vi "ExDriver.vi"(4 "Error In":errorcluster, 7 "Command":string) -> (0 "Error Out":errorcluster, 3 "Response":string)   [LabVIEW 2018]
uses:
  MOKO_LabViewLibrary/MokoLowLevel/MokoLowLovelControl/MLLC_DriverName.ctl
  MOKO_LabViewLibrary/MokoLowLevel/MokoLowLovelControl/MLLC_ConnectCluster.ctl
  MOKO_LabViewLibrary/MokoLowLevel/MokoLowLovelControl/MLLC_InterfaceType.ctl
  MOKO_LabViewLibrary/MokoLowLevel/MokoLowLovelControl/MLLC_OpenedSession.ctl
  MOKO_LabViewLibrary/MokoLowLevel/MokoLowLovelControl/MLLC_InterfaceSettings.ctl
  MOKO_LabViewLibrary/MokoLowLevel/MokoLowLovelControl/MLLC_InterfaceKind.ctl
  MOKO_LabViewLibrary/MokoLowLevel/MokoLowLovelControl/MLLC_Request.ctl
  MOKO_LabViewLibrary/MokoLowLevel/MokoLowLovelControl/MLLC_ResponseInit.ctl
panel:
  in  "Response Init":T1="43B"
  in  "Request":T2="ID"
  in  "Settings":T8={"Saved Data"=variant, "Data"={"Connect"={"InterfaceType"=enum."VISA", "OpenedSession"="", "InterfaceSettings"={"Interface"=enum."RS232", "EOS 4 read"=enum."LF (\\n)", "EOS 4 write"=enum."LF (\\n)", "TMO, ms"=10000, "Sett"=variant(cluster{"Baud Rate":u32, "Data Bits":u16, "Parity":u16, "Stop Bits":u16, "Flow Control":u16, "Eho":bool} {"Baud Rate"=75, "Data Bits"=0, "Parity"=0, "Stop Bits"=0, "Flow Control"=0, "Eho"=FALSE})}}, "Values"={"Value"=0.0}}}
  in  "Error Code":u32
  in  "Driver Name":T9="ExDriver"
  in  "Mode":T10(ring)
  # "ExDriver"
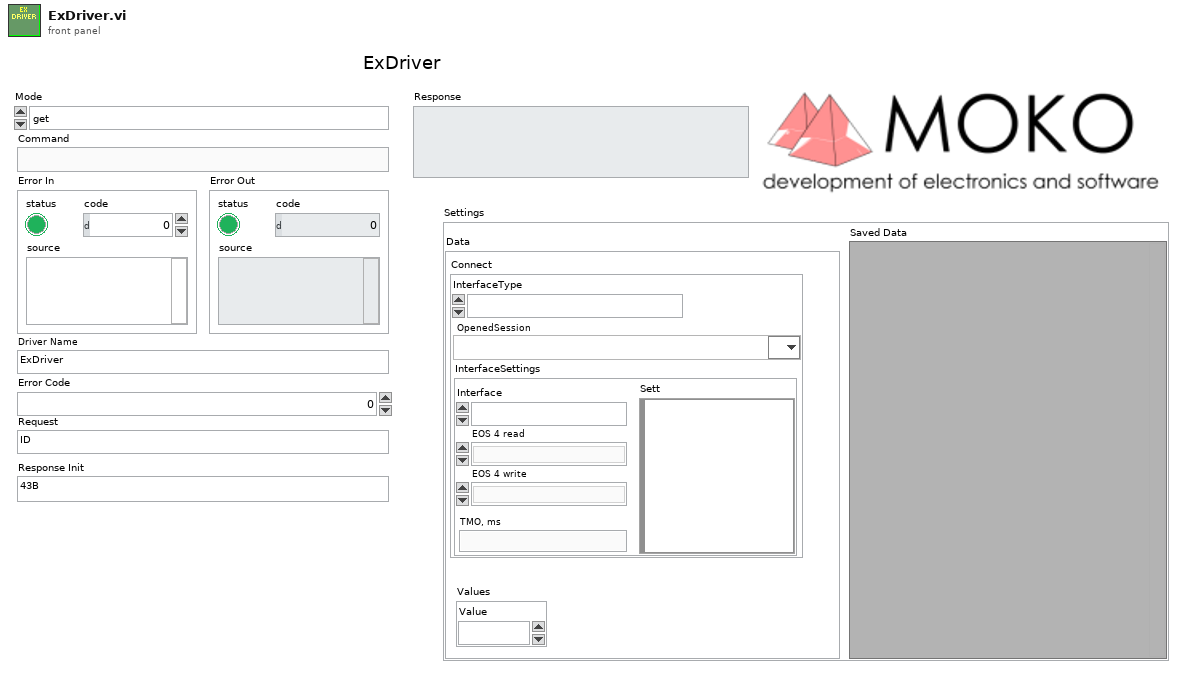
[diagram p1: front panel]
types:
  T1 = typedef "MLLC_ResponseInit.ctl" = string
  T2 = typedef "MLLC_Request.ctl" = string
  T3 = typedef "MLLC_ConnectCluster.ctl" = cluster{"InterfaceType":T4, "OpenedSession":T5, "InterfaceSettings":T6}
  T4 = typedef "MLLC_InterfaceType.ctl" = enum16{"VISA", "Prologix USB-GPIB"}
  T5 = typedef "MLLC_OpenedSession.ctl" = refnum<visa-resource-name>
  T6 = typedef "MLLC_InterfaceSettings.ctl" = cluster{"Interface":T7, "EOS 4 read":enum16{"Default (=EOS 4 write)", "CR (\\r)", "LF (\\n)", "None"}, "EOS 4 write":enum16{"CR+LF (\\r\\n)", "CR (\\r)", "LF (\\n)", "None"}, "TMO, ms":i32, "Sett":variant}
  T7 = typedef "MLLC_InterfaceKind.ctl" = enum16{"RS232", "GPIB", "USB", "Ethernet", "another"}
  T8 = cluster{"Saved Data":variant, "Data":cluster{"Connect":T3, "Values":cluster{"Value":dbl}}}
  T9 = typedef "MLLC_DriverName.ctl" = string
  T10 = enum16{"get", "set", "close", "Init", "Check", "ID"}
  T11 = cluster{"Connect":T3, "Values":cluster{"Value":dbl}}
  T12 = typedef "MLLC_Mode.ctl" = enum16{"get", "set", "close", "Init", "Check"}
  T13 = typedef "MLLC_Error.ctl" = errorcluster
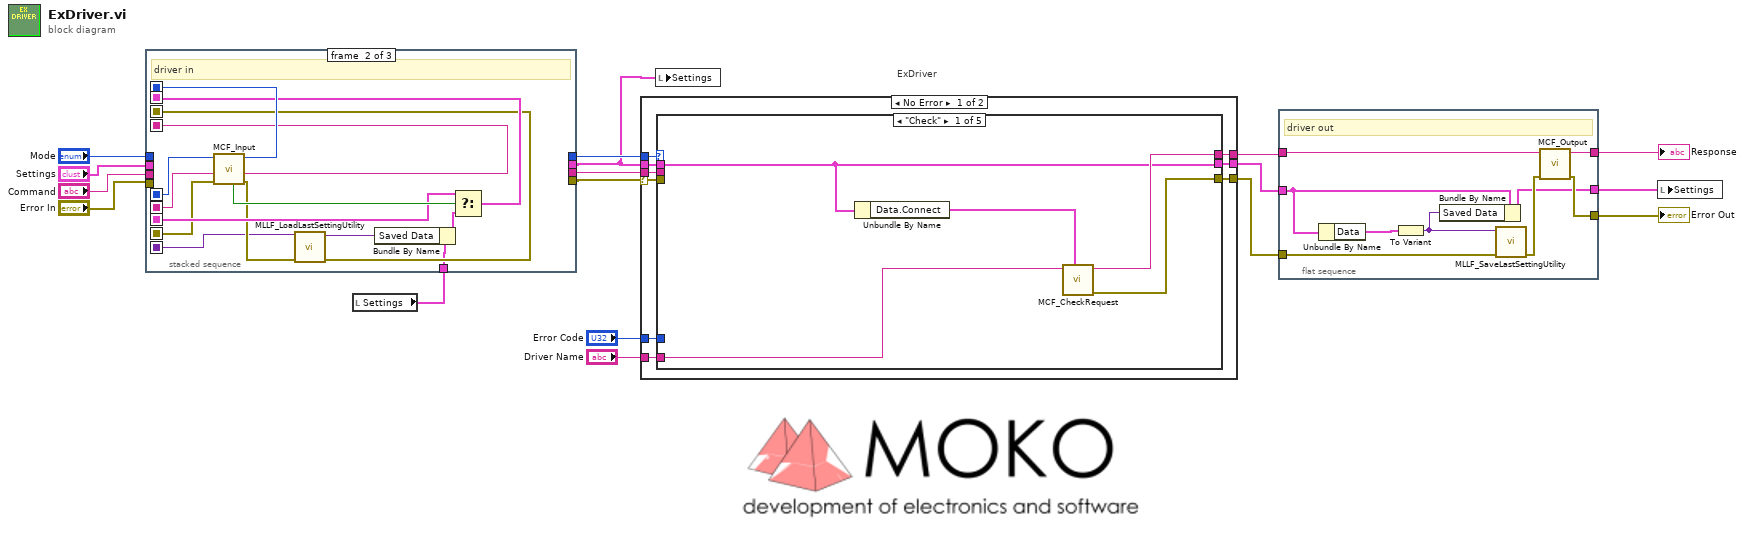
[diagram p0: block diagram]
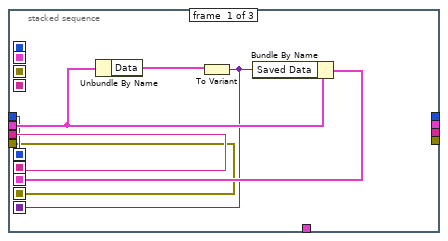
[diagram p2: hidden frame]
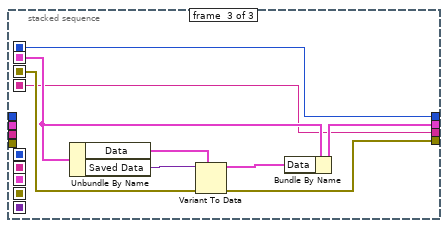
[diagram p3: hidden frame]
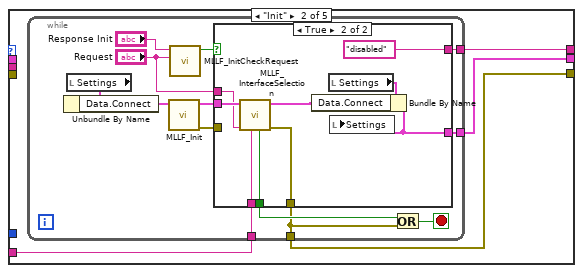
[diagram p4: hidden frame]
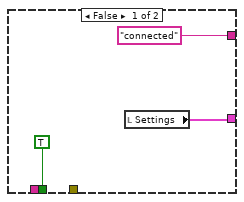
[diagram p5: hidden frame]
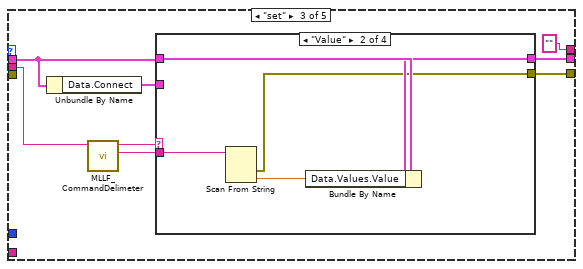
[diagram p6: hidden frame]
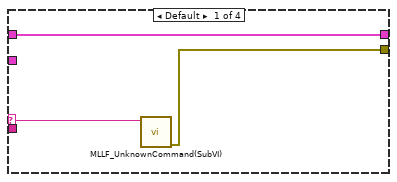
[diagram p7: hidden frame]
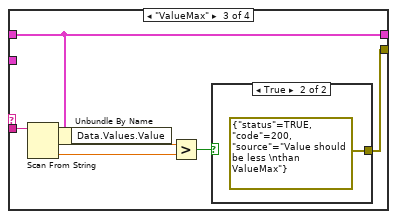
[diagram p8: hidden frame]
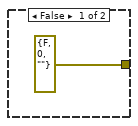
[diagram p9: hidden frame]
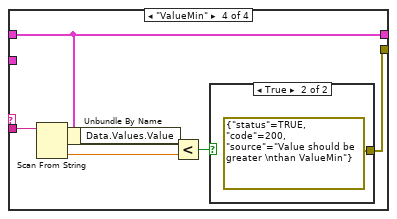
[diagram p10: hidden frame]
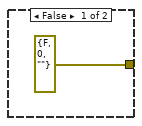
[diagram p11: hidden frame]
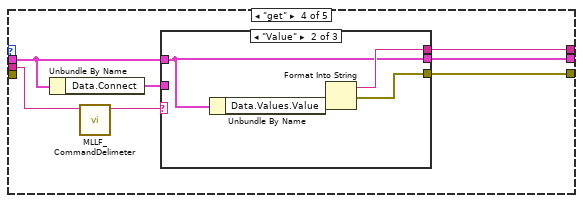
[diagram p12: hidden frame]
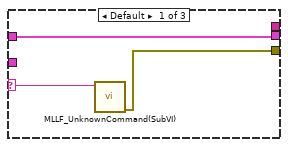
[diagram p13: hidden frame]
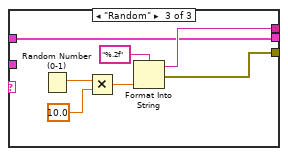
[diagram p14: hidden frame]
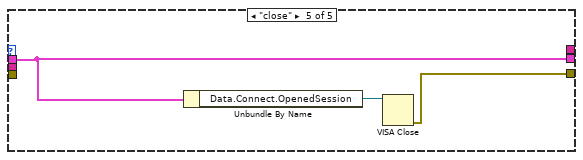
[diagram p15: hidden frame]
diagram:
  # "ExDriver"
  n1 = local read "Settings"() -> (w9:T8)
  n2 = stacked-sequence {
    seq-local: [w20 _ _] -> [_ w36 _]
    seq-local: [w19 _ _] -> [_ w37 _]
    seq-local: [w22 _ _] -> [_ w32 _]
    seq-local: [w18 _ _] -> [_ w31 _]
    seq-local: [w21 _ _] -> [_ w27 _]
    seq-local: [_ w28 _] -> [_ _ w44]
    seq-local: [_ w38 _] -> [_ _ w41]
    seq-local: [_ w35 _] -> [_ _ w40]
    seq-local: [_ w34 _] -> [_ _ w45]
    tunnel: "Command" -> [w20 _ _]
    tunnel: "Mode" -> [w19 _ _]
    tunnel: "Error In" -> [w18 _ _]
    tunnel: "Settings" -> [w23 _ _]
    tunnel: w9 -> [_ w26 _]
    tunnel: [_ _ w40] -> w5
    tunnel: [_ _ w43] -> w6
    tunnel: [_ _ w42] -> w4
    tunnel: [_ _ w41] -> w7
    frame #0 {
      n3 = Unbundle By Name(w23) -> ("Data"=w24:T11)
      n4 = To Variant(anything=w24) -> (Variant=w21:variant)
      n5 = Bundle By Name(cluster=w23, "Saved Data"=w21) -> (w22:T8)
    }
    frame #1 {
      # "driver in"
      n6 = call "MCF_Input.vi"("Error In"=w31, "Command in"=w36, "Mode in"=w37) -> ("Error Out"=w30:errorcluster, "Command out"=w35:string, "Mode out"=w38:T12, "Boolean"=w33:bool)  [unwired: 5 in]
      n7 = call "MLLF_LoadLastSettingUtility.vi"("Error In"=w30, "Save data in"=w27) -> ("Error Out"=w28:errorcluster, "Save data out"=w25:variant)  [unwired: 8 in]
      n8 = Bundle By Name(cluster=w26, "Saved Data"=w25) -> (w29:T8)
      n9 = Select(t=w32, s=w33, f=w29) -> (s? t:f=w34:T8)
    }
    frame #2 {
      n10 = Unbundle By Name(w45) -> ("Data"=w46:T11, "Saved Data"=w39:variant)
      n11 = Variant To Data(error in=w44, type=w46, Variant=w39) -> (data=w47:T11, error out=w42:errorcluster)
      n12 = Bundle By Name(cluster=w45, "Data"=w47) -> (w43:T8)
    }
  }
  n13 = case shown="No Error" w4 {
    selector: w4 -> [w52 w148]
    tunnel: [w54 w148] -> w13
    tunnel: w7 -> [w56 _]
    tunnel: [w55 _] -> w15
    tunnel: w5 -> [w53 _]
    tunnel: w6 -> [w49 w147]
    tunnel: "Error Code" -> [w51 _]
    tunnel: "Driver Name" -> [w50 _]
    tunnel: [w48 w147] -> w14
    frame No Error {
      n14 = case shown="\"Check\"" w56 {
        tunnel: [w60 w63 "" ("Output String") w123 _] -> w55
        tunnel: [w59 w65 w91 w124 w145] -> w54
        tunnel: w53 -> [_ _ w94 w126 _]
        tunnel: w52 -> [_ _ _ _ _]
        tunnel: w51 -> [_ _ _ _ _]
        tunnel: w50 -> [w61 w62 _ _ _]
        tunnel: w49 -> [w58 _ w98 w129 w144]
        tunnel: [w58 w64 w97 w128 w144] -> w48
        frame "Check" {
          # "Проверка подленности пользователя в соответствии с протоколом MD5."
          n15 = Unbundle By Name(w58) -> ("Data.Connect"=w57:T3)
          n16 = call "MCF_CheckRequest.vi"("Permanent data.Connect"=w57, "Driver Name"=w61) -> ("Error Out"=w59:errorcluster, "Output String"=w60:string)  [unwired: 8 in]
        }
        frame "Init" {
          # "Тут проходит инициализация оборудования"
          n17 = while {
            tunnel: [w77] -> w65
            tunnel: w62 -> [w70]
            tunnel: [w74] -> w64
            tunnel: [w71] -> w63
            stop <- w76 stop-if-true
            n18 = local read "Settings"() -> (w75:T8)
            n19 = Unbundle By Name(w75) -> ("Data.Connect"=w73:T3)
            n20 = call "MLLF_Init.vi"("DriverConnect in"=w73) -> ("Error Out"=w67:errorcluster, "DriverConnect out"=w72:T3)  [unwired: 7 in]
            n21 = call "MLLF_InitCheckRequest.vi"("Answer"="Request", "Response Init"="Response Init") -> ("Design"=w68:bool)  [unwired: 6 in, 3 out]
            n22 = case shown="True" w68 {
              tunnel: w72 -> [_ w89]
              tunnel: [TRUE w85] -> w78
              tunnel: [_ w90] -> w77
              tunnel: [w80 w86] -> w74
              tunnel: ["connected" "disabled"] -> w71
              tunnel: w70 -> [_ w83]
              tunnel: w67 -> [_ _]
              tunnel: "Request" -> [_ w82]
              frame False {
                n23 = local read "Settings"() -> (w80:T8)
              }
              frame True {
                n24 = call "MLLF_InterfaceSelection.vi"("Driver Name"=w83, "Answer:"=w82, "DriverConnect in"=w89) -> ("error out"=w90:T13, "DriverConnect out"=w88:T3, "stop init?"=w85:bool)  [unwired: 4 in, 2 out]
                n25 = local read "Settings"() -> (w87:T8)
                n26 = Bundle By Name(cluster=w87, "Data.Connect"=w88) -> (w86:T8)
                n27 = local write "Settings"(w86) -> ()
              }
            }
            n28 = Or(x=w78, y=w77) -> (x .or. y?=w76:bool)
          }
        }
        frame "set" {
          # "Тут реализованы функции DriverSet"
          n29 = Unbundle By Name(w98) -> ("Data.Connect"=w95:T3)
          n30 = call "MLLF_CommandDelimeter.vi"("command with param"=w94) -> ("param 1"=w92:string, "command"=w93:string)  [unwired: 6 in, 3 out]
          n31 = case shown="\"Value\"" w93 {
            selector: w93 -> [w100 _ _ _]
            tunnel: [w101 w103 w107 w115] -> w97
            tunnel: w98 -> [w101 w106 w107 w115]
            tunnel: w95 -> [_ _ _ _]
            tunnel: w92 -> [_ w105 w112 w120]
            tunnel: [w99 w102 w108 w116] -> w91
            frame Default {
              n32 = call "MLLF_UnknownCommand(SubVI).vi"("Unknown command"=w100) -> ("error out"=w99:errorcluster)  [unwired: 10 in]
            }
            frame "Value" {
              n33 = Scan From String(input string=w105) -> (error out=w102:errorcluster, output 1=w104:dbl)  [unwired: 4 in, 2 out]
              n34 = Bundle By Name(cluster=w106, "Data.Values.Value"=w104) -> (w103:T8)
            }
            frame "ValueMax" {
              n35 = Scan From String(input string=w112) -> (output 1=w111:dbl)  [unwired: 4 in, 3 out]
              n36 = Unbundle By Name(w107) -> ("Data.Values.Value"=w110:dbl)
              n37 = Greater?(x=w110, y=w111) -> (0:w109:bool)
              n38 = case shown="True" w109 {
                tunnel: [errorcluster {"status"=FALSE, "code"=0, "source"=""} ("error IO") errorcluster {"status"=TRUE, "code"=200, "source"="Value should be less \nthan ValueMax"} ("error IO")] -> w108
                frame False {
                }
                frame True {
                }
              }
            }
            frame "ValueMin" {
              n39 = Scan From String(input string=w120) -> (output 1=w119:dbl)  [unwired: 4 in, 3 out]
              n40 = Unbundle By Name(w115) -> ("Data.Values.Value"=w118:dbl)
              n41 = Less?(x=w118, y=w119) -> (x < y?=w117:bool)
              n42 = case shown="True" w117 {
                tunnel: [errorcluster {"status"=FALSE, "code"=0, "source"=""} ("error IO") errorcluster {"status"=TRUE, "code"=200, "source"="Value should be greater \nthan ValueMin"} ("error IO")] -> w116
                frame False {
                }
                frame True {
                }
              }
            }
          }
        }
        frame "get" {
          # "Тут реализованы функции DriverGet"
          n43 = Unbundle By Name(w129) -> ("Data.Connect"=w127:T3)
          n44 = call "MLLF_CommandDelimeter.vi"("command with param"=w126) -> ("command"=w125:string)  [unwired: 6 in, 4 out]
          n45 = case shown="\"Value\"" w125 {
            selector: w125 -> [w131 _ _]
            tunnel: w127 -> [_ _ _]
            tunnel: w129 -> [w132 w134 w142]
            tunnel: [w132 w134 w142] -> w128
            tunnel: [w130 w133 w137] -> w124
            tunnel: [_ w135 w143] -> w123
            frame Default {
              n46 = call "MLLF_UnknownCommand(SubVI).vi"("Unknown command"=w131) -> ("error out"=w130:errorcluster)  [unwired: 10 in]
            }
            frame "Value" {
              n47 = Unbundle By Name(w134) -> ("Data.Values.Value"=w136:dbl)
              n48 = Format Into String(w136) -> (resulting string=w135:string, error out=w133:errorcluster)  [unwired: 3 in]
            }
            frame "Random" {
              n49 = Random Number (0-1)() -> (number: 0 to 1=w141:dbl)
              n50 = Multiply(x=w141, y=10.0) -> (x*y=w139:dbl)
              n51 = Format Into String(format string="%.2f", w139) -> (resulting string=w143:string, error out=w137:errorcluster)  [unwired: 2 in]
            }
          }
        }
        frame "close" {
          # "Завершение сессии"
          n52 = Unbundle By Name(w144) -> ("Data.Connect.OpenedSession"=w146:T5)
          n53 = VISA Close(VISA resource name=w146) -> (error out=w145:errorcluster)  [unwired: 1 in]
        }
      }
    }
    frame Error {
    }
  }
  n54 = local write "Settings"(w6) -> ()
  n55 = flat-sequence {
    tunnel: [w157] -> w11
    tunnel: [w156] -> w12
    tunnel: w15 -> [w155]
    tunnel: w13 -> [w154]
    tunnel: w14 -> [w150]
    tunnel: [w152] -> w10
    frame #0 {
      # "driver out"
      n56 = Unbundle By Name(w150) -> ("Data"=w149:T11)
      n57 = To Variant(anything=w149) -> (Variant=w151:variant)
      n58 = Bundle By Name(cluster=w150, "Saved Data"=w151) -> (w152:T8)
      n59 = call "MLLF_SaveLastSettingUtility.vi"("error in"=w154, "Saved Data"=w151) -> ("error out"=w153:T13)  [unwired: 8 in, 1 out]
      n60 = call "MCF_Output.vi"("Error In"=w153, "Input"=w155) -> ("Error Out"=w156:errorcluster, "Output"=w157:string)  [unwired: 8 in]
    }
  }
  n61 = local write "Settings"(w10) -> ()
  "Response" <- w11
  "Error Out" <- w12
